vi "Create New Document.vi"(8 "error in (no error)":errorcluster, 11 "File Path":path) -> (0 "error out":errorcluster, 3 "Document out":refnum<class "Document.lvclass">)   [LabVIEW 2017, in "LabVIEW NPOI.lvlib" / "Document.lvclass"]
doc: "Creates a new <b>Document</b> at the <b>File Path</b> location. Use save to persist your changes.\n\nNotes:\n - If <b>File Path</b> is empty (default) or is <Not A Path> or is a directory, the VI displays a dialog box from which the user can select a file. Error 43 occurs if you cancel the dialog box. \n - If the <b>File Path</b> already contains a docuement with the same name then that file is overwritten without warning."
uses:
  Document.lvclass
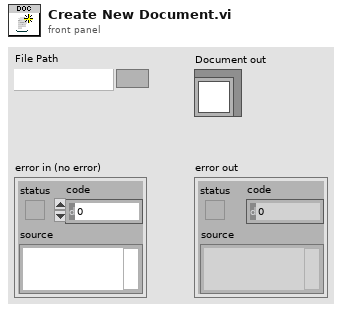
[diagram p1: front panel]
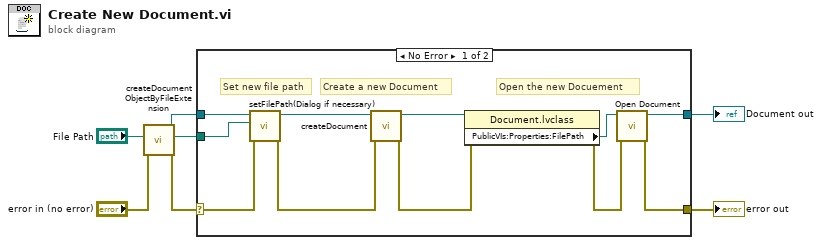
[diagram p0: block diagram]
diagram:
  n1 = call "createDocumentObjectByFileExtension.vi"("error in (no error)"="error in (no error)", "File Path"="File Path") -> ("error out"=w2:errorcluster, "File Path dup"=w4:path, "Document out"=w3:refnum<class "Document.lvclass">)  [unwired: 7 in]
  n2 = case shown="No Error" w2 {
    selector: w2 -> [w10 w20]
    tunnel: [w17 w20] -> w7
    tunnel: [w18 w19] -> w6
    tunnel: w3 -> [w15 w19]
    tunnel: w4 -> [w9 _]
    frame No Error {
      # "Create a new Document"
      # "Set new file path"
      # "Open the new Docuement"
      n3 = call "setFilePath(Dialog if necessary).vi"("error in (no error)"=w10, "FilePath"=w9, "Document in"=w15) -> ("error out"=w13:errorcluster, "Document out"=w14:refnum<class "Document.lvclass">)  [unwired: 7 in]
      n4 = call-dynamic "createDocument.vi"("error in (no error)"=w13, "Document in"=w14) -> ("error out"=w12:errorcluster, "Document out"=w16:refnum<class "Document.lvclass">)  [unwired: 8 in]
      n5 = property class="Document.lvclass"(reference=w16, error in=w12) -> (error out=w11:errorcluster, "PublicVIs:Properties:FilePath"=w8:path)  [unwired: 1 out]
      n6 = call "Open Document.vi"("error in (no error)"=w11, "File Path"=w8) -> ("error out"=w17:errorcluster, "Document out"=w18:refnum<class "Document.lvclass">)  [unwired: 8 in]
    }
    frame Error {
    }
  }
  "error out" <- w7
  "Document out" <- w6
